vi "4 probe data-osc-time v1.7 not mean contionus.vi"() -> ()   [LabVIEW 2014]
uses:
  <vilib>/Analysis/baseanly.llb/Mean (DBL).vi
  <instrlib>/Tektronix TDS 200 1000 2000 Series/Tektronix TDS 200 1000 2000 Series.lvlib
  <vilib>/Analysis/NI_AALBase.lvlib
panel:
  out "Osc. Ch.1 Data":string
  in  "Osc. Ch.1 Data 2":path=path "c:/myfile.txt"
  out "Ch1":dbl
  in  "loop num":dbl=10000000000.0
  in  "stop button":bool
  out "Seconds":sgl
  out "Chamber *C Graph":dbl(graph)
  in  "Channel 1 (0: Channel 1)":u16(ring) items=["Channel 1", "Channel 2", "Channel 3", "Channel 4", "Math", "Reference A", "Reference B", "Reference C", "Reference D"]
  in  "Serial Configuration":T1={"Baud Rate"=9600, "Parity"=0, "Stop Bits"=10, "Flow Control"=2} {"Flow Control" items=["None", "XON/XOFF", "RTS/CTS", "XON/XOFF & RTS/CTS", "DTR/DSR", "XON/XOFF & DTR/DSR"]; "Stop Bits" items=["1.0"=10, "1.5"=15, "2.0"=20]; "Parity" items=["None", "Odd", "Even", "Mark", "Space"]; "Baud Rate" items=["300"=300, "600"=600, "1200"=1200, "2400"=2400, "4800"=4800, "9600"=9600, "19200"=19200]}
  in  "Probe Attenuation 1 (0.1)":dbl=0.1
  in  "Vertical Coupling 1 (1: DC)":u16(ring)=1 items=["AC", "DC", "Ground"]
  in  "Timeout (10000 ms)":u32=500
  in  "VISA resource name":refnum<visa-resource-name>="USB0::0x0699::0x03A6::C044157::INSTR"
  in  "Start Button":bool
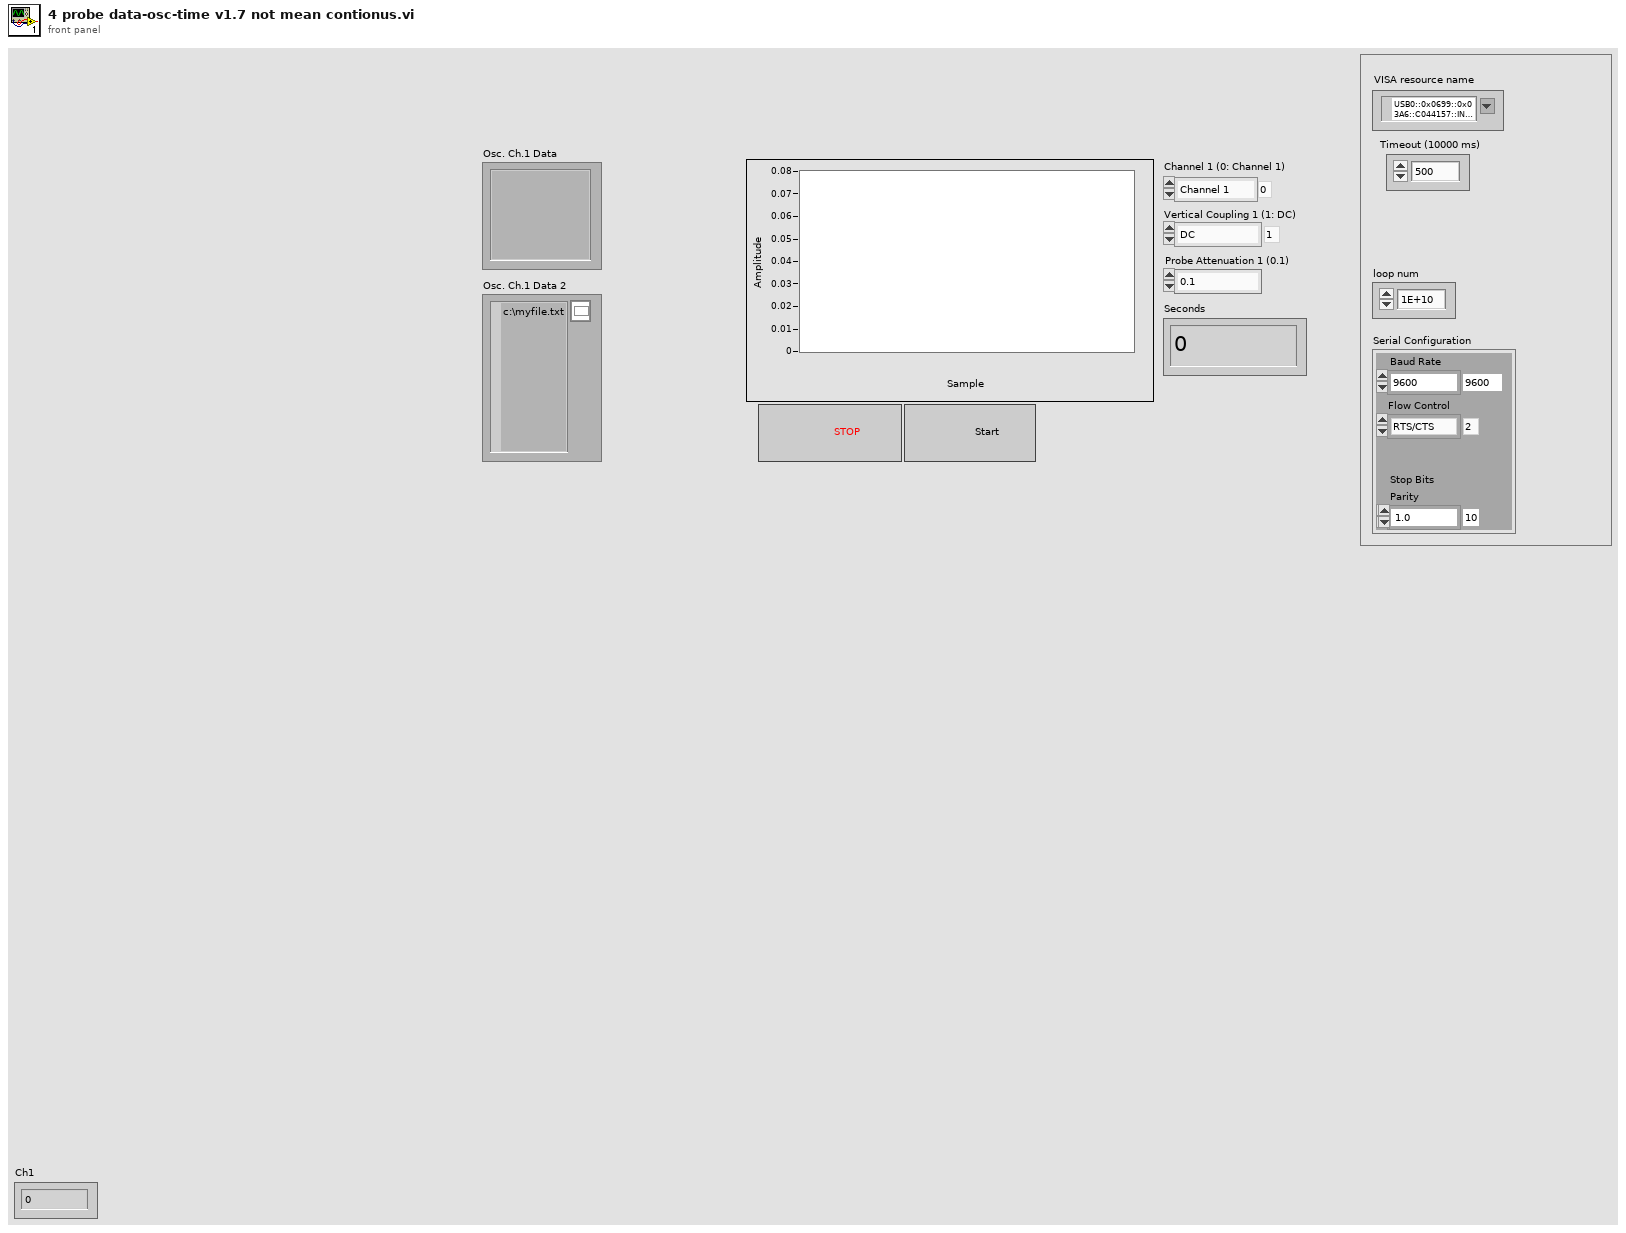
[diagram p1: front panel]
types:
  T1 = cluster{"Baud Rate":u32, "Parity":u16, "Stop Bits":u16, "Flow Control":u16}
  T2 = enum16{"open", "replace", "create", "open or create", "replace or create", "replace or create with confirmation"}
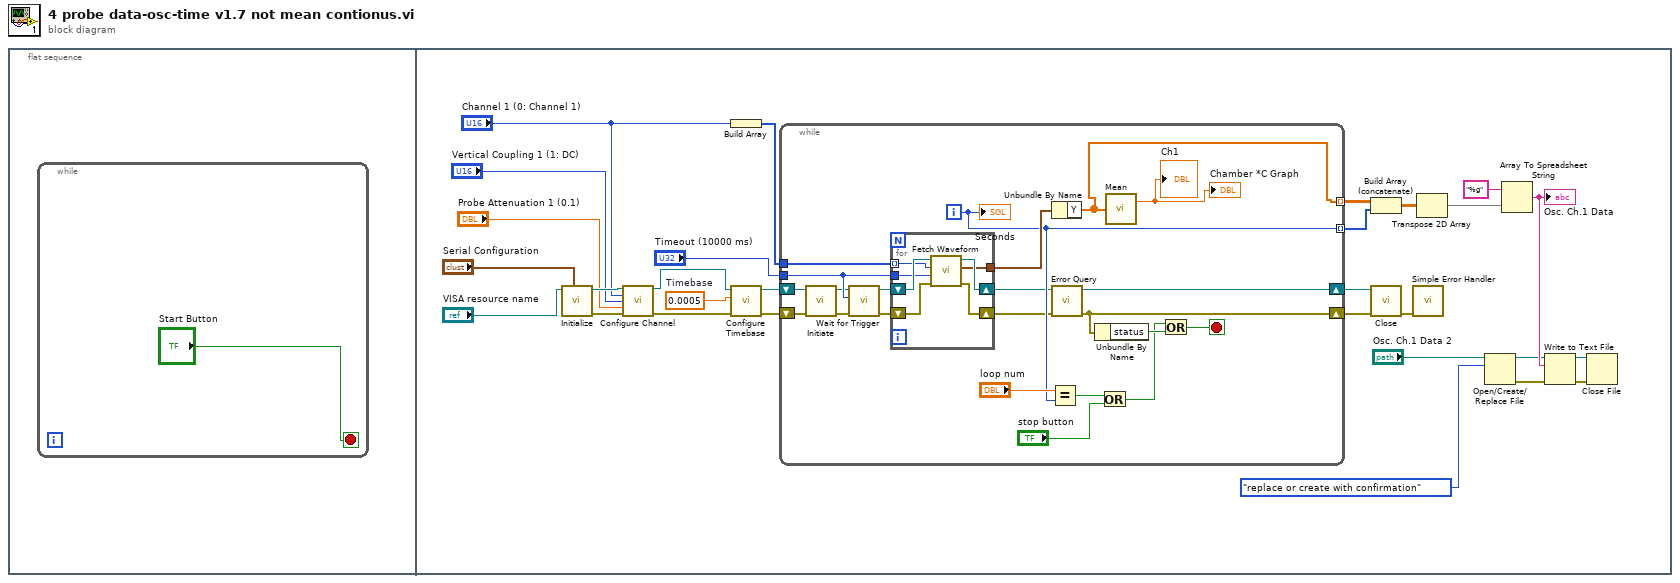
[diagram p0: block diagram]
diagram:
  n1 = flat-sequence {
    frame #0 {
      n2 = while {
        stop <- "Start Button" stop-if-true
      }
    }
    frame #1 {
      w20 = 0.0005  # Timebase
      n3 = call <instrlib>:"Initialize.vi"("Serial Configuration"="Serial Configuration", "VISA resource name"="VISA resource name") -> ("error out"=w25:errorcluster, "VISA resource name out"=w26:refnum<visa-resource-name>)  [unwired: 3 in, 5 out]
      n4 = call <instrlib>:"Configure Channel.vi"("VISA resource name"=w26, "Channel (0: Channel 1)"="Channel 1 (0: Channel 1)", "Vertical Coupling (1: DC)"="Vertical Coupling 1 (1: DC)", "Probe Attenuation (10: 10X)"="Probe Attenuation 1 (0.1)", "error in (no error)"=w25) -> ("VISA resource name out"=w5:refnum<visa-resource-name>, "error out"=w4:errorcluster)  [unwired: 4 in, 5 out]
      n5 = Build Array("Channel 1 (0: Channel 1)") -> (w19:u16[])
      n6 = call <instrlib>:"Configure Timebase.vi"("error in (no error)"=w4, "Timebase (0.0005 s)"=w20, "VISA resource name"=w5) -> ("error out"=w23:errorcluster, "VISA resource name out"=w24:refnum<visa-resource-name>)  [unwired: 1 in, 6 out]
      n7 = while {
        tunnel: w19 -> [w49]
        tunnel: "Timeout (10000 ms)" -> [w48]
        shift-right: [w52] -> w28
        shift-left: w24 -> [w51]
        shift-right: [w37] -> w27
        shift-left: w23 -> [w50]
        tunnel: [w36] -> w2 mode=indexing
        tunnel: [w31] -> w3 mode=indexing
        i -> [w36]
        stop <- w35 stop-if-true
        n8 = call <instrlib>:"Initiate.vi"("error in (no error)"=w50, "VISA resource name"=w51) -> ("error out"=w44:errorcluster, "VISA resource name out"=w47:refnum<visa-resource-name>)  [unwired: 8 out]
        n9 = call <instrlib>:"Wait for Trigger.vi"("error in (no error)"=w44, "Timeout (10000 ms)"=w48, "VISA resource name"=w47) -> ("error out"=w45:errorcluster, "VISA resource name out"=w46:refnum<visa-resource-name>)  [unwired: 7 out]
        n10 = for {
          shift-right: [w58] -> w33
          shift-left: w45 -> [w56]
          tunnel: w49 -> [w54] mode=indexing
          tunnel: w48 -> [w55]
          shift-right: [w59] -> w34
          shift-left: w46 -> [w57]
          tunnel: [w53] -> w43
          n11 = call <instrlib>:"Fetch Waveform.vi"("error in (no error)"=w56, "Timeout (10000 ms)"=w55, "Source (0: Channel 1)"=w54, "VISA resource name"=w57) -> ("error out"=w58:errorcluster, "Waveform Data"=w53:waveform(dbl), "VISA resource name out"=w59:refnum<visa-resource-name>)  [unwired: 2 in, 3 out]
        }
        n12 = Equal?(x="loop num", y=w36) -> (x = y?=w38:bool)
        n13 = Unbundle By Name(w43) -> ("Y"=w31:dbl[])
        n14 = call <instrlib>:"Error Query.vi"("error in (no error)"=w33, "VISA resource name"=w34) -> ("error out"=w37:errorcluster, "VISA resource name out"=w52:refnum<visa-resource-name>)  [unwired: 8 out]
        n15 = Unbundle By Name(w37) -> ("status"=w40:bool)
        n16 = Or(x=w38, y="stop button") -> (x .or. y?=w39:bool)
        n17 = call-poly <vilib>:"Mean.vi"("X"=w31) -> ("mean"=→"Ch1" →"Chamber *C Graph":dbl)  [unwired: 1 out]
        n18 = Or(x=w39, y=w40) -> (x .or. y?=w35:bool)
        "Seconds" <- w36
      }
      n19 = Build Array (concatenate)(w3, w2) -> (w13:dbl[][])
      n20 = call <instrlib>:"Close.vi"("error in (no error)"=w27, "VISA resource name"=w28) -> ("error out"=w29:errorcluster)  [unwired: 9 out]
      n21 = call <vilib>:"Simple Error Handler.vi"("error in (no error)"=w29) -> ()  [unwired: 1 in, 8 out]
      n22 = Transpose 2D Array(2D array=w13) -> (transposed array=w15:dbl[][])
      n23 = Open/Create/Replace File(file path (use dialog)="Osc. Ch.1 Data 2", operation (0:open)=T2."replace or create with confirmation") -> (refnum out=w12:refnum<file>, error out=w7:errorcluster)  [unwired: 4 in, 1 out]
      n24 = Array To Spreadsheet String(array=w15, 3:"%g" ("format string")) -> (spreadsheet string=w16:string)  [unwired: 1 in]
      "Osc. Ch.1 Data" <- w16
      n25 = Write to Text File(file (use dialog)=w12, text=w16, error in=w7) -> (refnum out=w9:refnum<file>, error out=w8:errorcluster)  [unwired: 2 out]
      n26 = Close File(refnum=w9, error in=w8) -> ()  [unwired: 2 out]
    }
  }
